vi "Cell Details.vi"(8 "error in (no error)":errorcluster, 10 "Cell, Alignment, LS and Font":T1={"Text"={"Cell Alignment"=0, "Text rotation"=enum."None", "Line spacing"=enum."1.0"}, "Cell Appearance"={"Border"=0, "Thickness"=0.5, "Color"=0, "BG"=16777225}, "HMerge"={"From"=-1, "to"=-1}, "VMerge"={"From"=-1, "to"=-1}, "Font"={"Name"="", "Size"=0.0, "Color"=0, "Style"={"Bold"=FALSE, "Italic"=FALSE, "Underline"=FALSE, "Strikeout"=FALSE}, "Type"={"Type&direction"=enum."Select", "Embedded"=FALSE, "Encoding"=""}}}, 11 "PDF Report":refnum<class "PDF Report Class.lvclass">) -> (0 "error out":errorcluster, 2 "Cell Cluster":T15={"Font Ref"=refnum, "Close font ref"=FALSE, "Type and run direction"=enum."Select", "Cell Alignment"=0, "Text rotation"=enum."None", "Leading"=18.0, "PdfP Cell ref"=refnum, "Colspan"=-1}, 3 "PDF Report duplicate":refnum<class "PDF Report Class.lvclass">)   [LabVIEW 2019, in "Exaprom PDF.lvlib"]
doc: "Version 1.0\nDeveloped by Jean-Marc Simard\nCopyright © 2010, Exaprom Inc.\nAll rights reserved.\nLicense: BSD\n\nWith iTextSharp 4.1.6 (http://itextsharp.sourceforge.net)\nunder Mozilla Public License Version 1.1\n(http://www.mozilla.org/MPL/MPL-1.1.html)"
uses:
  Exaprom PDF.lvlib
  Controls/Table Controls/Cell Cluster.ctl
  C:/work/niobrara_lv/labview pdf writer fixing/DLL/itextsharp.dll
  DLL/itextsharp.dll
  Controls/Text Controls/Unicode/Type and run direction.ctl
  Controls/Table Controls/Cell Alignment 20px.ctl
  Controls/Table Controls/Text vertical arrangement.ctl
  Controls/Font Controls/Font size.ctl
  LV Class/PDF Report Class/PDF Report Class.lvclass
  Controls/Table Controls/Cell, Alignment, LS and Font.ctl
  Controls/Table Controls/Cell Type, Alignment and LS.ctl
  Controls/Text Controls/Line spacing.ctl
  Controls/Table Controls/Cell Appearance.ctl
  Controls/Table Controls/Cell Border 20 px.ctl
  Controls/Table Controls/Merge Horizontal.ctl
  Controls/Table Controls/Merge Vertical.ctl
  Controls/Font Controls/Font complete cluster.ctl
  Controls/Font Controls/Font color.ctl
  Controls/Font Controls/Type and encoding.ctl
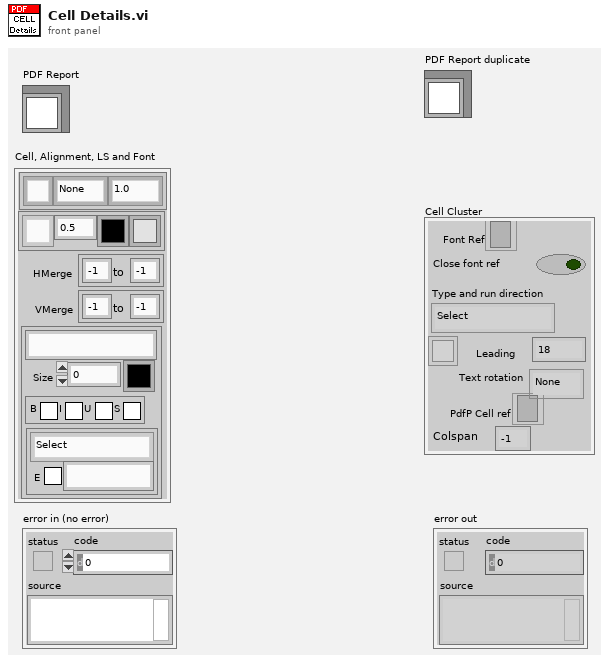
[diagram p1: front panel]
types:
  T1 = typedef "Exaprom PDF.lvlib/Cell, Alignment, LS and Font.ctl" = cluster{"Text":T2, "Cell Appearance":T6, "HMerge":T8, "VMerge":T9, "Font":T10}
  T2 = typedef "Exaprom PDF.lvlib/Cell Type, Alignment and LS.ctl" = cluster{"Cell Alignment":T3, "Text rotation":T4, "Line spacing":T5}
  T3 = typedef "Exaprom PDF.lvlib/Cell Alignment 20px.ctl" = u16
  T4 = typedef "Exaprom PDF.lvlib/Text vertical arrangement.ctl" = enum16{"None", "Clockwise", "Counterclockwise"}
  T5 = typedef "Exaprom PDF.lvlib/Line spacing.ctl" = enum16{"Select", "1.0", "1.5", "2.0"}
  T6 = typedef "Exaprom PDF.lvlib/Cell Appearance.ctl" = cluster{"Border":T7, "Thickness":sgl, "Color":u32, "BG":u32}
  T7 = typedef "Exaprom PDF.lvlib/Cell Border 20 px.ctl" = u16
  T8 = typedef "Exaprom PDF.lvlib/Merge Horizontal.ctl" = cluster{"From":i8, "to":i8}
  T9 = typedef "Exaprom PDF.lvlib/Merge Vertical.ctl" = cluster{"From":i8, "to":i8}
  T10 = typedef "Exaprom PDF.lvlib/Font complete cluster.ctl" = cluster{"Name":string, "Size":T11, "Color":T12, "Style":cluster{"Bold":bool, "Italic":bool, "Underline":bool, "Strikeout":bool}, "Type":T13}
  T11 = typedef "Exaprom PDF.lvlib/Font size.ctl" = sgl
  T12 = typedef "Exaprom PDF.lvlib/Font color.ctl" = u32
  T13 = typedef "Exaprom PDF.lvlib/Type and encoding.ctl" = cluster{"Type&direction":T14, "Embedded":bool, "Encoding":string}
  T14 = typedef "Exaprom PDF.lvlib/Type and run direction.ctl" = enum16{"Select", "ASCII", "UTF-16", "UTF-16 (default)", "UTF-16 (LTR)", "UTF-16 (RTL)"}
  T15 = typedef "Exaprom PDF.lvlib/Cell Cluster.ctl" = cluster{"Font Ref":refnum<k24>, "Close font ref":bool, "Type and run direction":T14, "Cell Alignment":T3, "Text rotation":T4, "Leading":T11, "PdfP Cell ref":refnum<k24>, "Colspan":i8}
  T16 = typedef "Exaprom PDF.lvlib/Texte alignement.ctl" = enum16{"Select", "CENTER", "JUSTIFY", "LEFT", "RIGHT"}
  T17 = typedef "Exaprom PDF.lvlib/Cell Vertical alignment.ctl" = enum16{"TOP", "MIDDLE", "BOTTOM"}
  T18 = cluster{"Horizontal Alignment":T16, "Line spacing":T5}
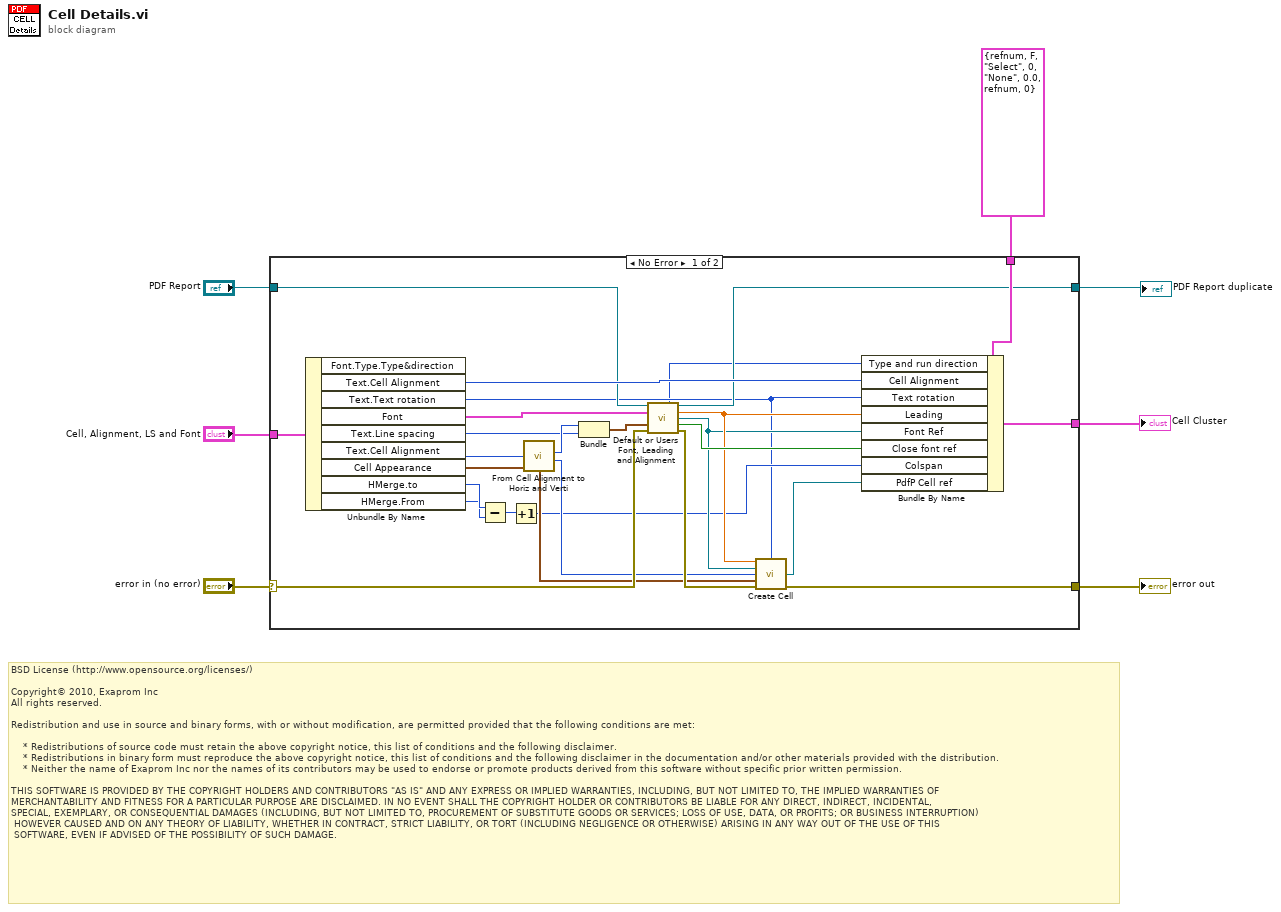
[diagram p0: block diagram]
diagram:
  # "BSD License (http://www.opensource.org/licenses/)\n\nCopyright© 2010, Exaprom Inc\nAll rights reserved.\n\nRedistribution and use in source and binary forms, with or without modification, are permitted provided that the following conditions are met:\n\n    * Redistributions of source code must retain the above copyright notice, this list of conditions and the following disclaimer.\n    * Redistributions in binary form must reproduce the above copyright notice, this list of conditions and the following disclaimer in the documentation and/or other materials provided with the distribution.\n    * Neither the name of Exaprom Inc nor the names of its contributors may be used to endorse or promote products derived from this software without specific prior written permission.\n\nTHIS SOFTWARE IS PROVIDED BY THE COPYRIGHT HOLDERS AND CONTRIBUTORS \"AS IS\" AND ANY EXPRESS OR IMPLIED WARRANTIES, INCLUDING, BUT NOT LIMITED TO, THE IMPLIED WARRANTIES OF \nMERCHANTABILITY AND FITNESS FOR A PARTICULAR PURPOSE ARE DISCLAIMED. IN NO EVENT SHALL THE COPYRIGHT HOLDER OR CONTRIBUTORS BE LIABLE FOR ANY DIRECT, INDIRECT, INCIDENTAL,\nSPECIAL, EXEMPLARY, OR CONSEQUENTIAL DAMAGES (INCLUDING, BUT NOT LIMITED TO, PROCUREMENT OF SUBSTITUTE GOODS OR SERVICES; LOSS OF USE, DATA, OR PROFITS; OR BUSINESS INTERRUPTION)\n HOWEVER CAUSED AND ON ANY THEORY OF LIABILITY, WHETHER IN CONTRACT, STRICT LIABILITY, OR TORT (INCLUDING NEGLIGENCE OR OTHERWISE) ARISING IN ANY WAY OUT OF THE USE OF THIS\n SOFTWARE, EVEN IF ADVISED OF THE POSSIBILITY OF SUCH DAMAGE."
  n1 = case shown="No Error" "error in (no error)" {
    selector: "error in (no error)" -> [w29 w36]
    tunnel: "Cell, Alignment, LS and Font" -> [w32 _]
    tunnel: T15 {"Font Ref"=refnum, "Close font ref"=FALSE, "Type and run direction"=enum."Select", "Cell Alignment"=0, "Text rotation"=enum."None", "Leading"=0.0, "PdfP Cell ref"=refnum, "Colspan"=0} ("Cell Cluster") -> [w31 w35]
    tunnel: [w30 w35] -> w7
    tunnel: [w19 w36] -> w6
    tunnel: "PDF Report" -> [w25 w34]
    tunnel: [w24 w34] -> w2
    frame No Error {
      n2 = Unbundle By Name(w32) -> ("Text.Cell Alignment"=w28:T3, "Text.Text rotation"=w9:T4, "Font"=w26:T10, "Text.Line spacing"=w21:T5, "Text.Cell Alignment"=w23:T3, "Cell Appearance"=w15:T6, "HMerge.to"=w14:i8, "HMerge.From"=w13:i8)  [unwired: 1 out]
      n3 = Subtract(x=w14, y=w13) -> (x-y=w12:i8)
      n4 = Increment(x=w12) -> (x+1=w11:i8)
      n5 = call "From Cell Alignment to Horiz and Verti.vi"("Cell Alignment"=w23) -> ("Horizontal Alignment"=w22:T16, "Vertical Alignement"=w16:T17)  [unwired: 6 in]
      n6 = Bundle("Horizontal Alignment"=w22, "Line spacing"=w21) -> (w33:T18)  [unwired: 1 out]
      n7 = call "Default or Users Font, Leading and Alignment.vi"("PDF Report"=w25, "Font"=w26, "Paragraphe cluster"=w33, "error in (no error)"=w29) -> ("Type and run direction"=w8:T14, "PDF Report duplicate"=w24:refnum<class "PDF Report Class.lvclass">, "Leading"=w18:T11, "Font Ref"=w17:refnum<k24>, "Close Font Ref"=w27:bool, "error out"=w20:errorcluster)  [unwired: 6 out]
      n8 = call "Create Cell.vi"("Leading"=w18, "Text rotation"=w9, "Font Ref"=w17, "Vertical Alignement"=w16, "Cell Appearance"=w15, "error in (no error)"=w20) -> ("PdfP Cell ref"=w10:refnum<k24>, "error out"=w19:errorcluster)  [unwired: 8 in]
      n9 = Bundle By Name(cluster=w31, "Type and run direction"=w8, "Cell Alignment"=w28, "Text rotation"=w9, "Leading"=w18, "Font Ref"=w17, "Close font ref"=w27, "Colspan"=w11, "PdfP Cell ref"=w10) -> (w30:T15)
    }
    frame Error {
    }
  }
  "Cell Cluster" <- w7
  "error out" <- w6
  "PDF Report duplicate" <- w2
